vi "Force Channel Command.vi"(8 "error in":errorcluster, 10 "Channel Force Data":T1 {"Force Data" format="%x"}, 11 "CoreOOB_Rx in":refnum<class "CIFCoreOOB_Rx.lvclass">) -> (0 "error out":errorcluster, 3 "CoreOOB_Rx out":refnum<class "CIFCoreOOB_Rx.lvclass">)   [LabVIEW 2021, in "CIFCoreOOB_Rx.lvclass"]
uses:
  CIFCoreOOB_Rx.lvclass
  D:/dev/CIF-LVCore/src/CIFUtilities/CIFOutOfBand/CIFOutOfBand.lvclass
  Typedef/Channel Fault Data.ctl
  CIFUtilities/CIFOutOfBand/CIFOutOfBand.lvclass/CIFOutOfBand.ctl
  Typedef/OOB Core Commands.ctl
  Typedef/Template Payload.ctl
  Typedef/Channel Connection Data.ctl
  CIFCoreOOB_Rx.lvclass/CIFCoreOOB_Rx.ctl
  CIFUtilities/CIFOutOfBand/CIFOutOfBand.lvclass
  <vilib>/CIF Foundation/CIF Utilities/Time/Typedef/Timestamp Pair.ctl
  <vilib>/CIF Foundation/CIF Utilities/Time/Time_CIF_U.lvlib
  <vilib>/CIF Foundation/CIF Utilities/Time/Typedef/Clock Conversion Map.ctl
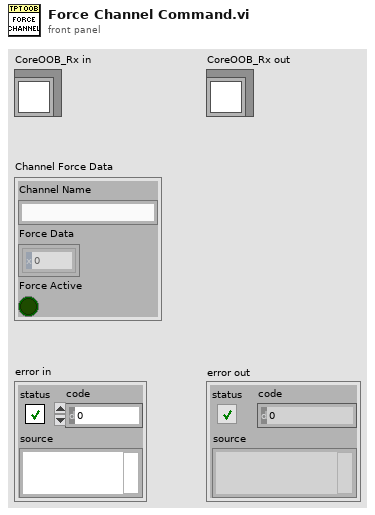
[diagram p1: front panel]
types:
  T1 = typedef "CIFCoreOOB_Rx.lvclass/Channel Fault Data.ctl" = cluster{"Channel Name":string, "Force Data":u8[], "Force Active":bool}
  T2 = typedef "CIFCoreOOB_Rx.lvclass/OOB Core Commands.ctl" = enum8{"Start", "Pause", "Stop", "RefreshStats", "UpdateConfig", "Connect Channel", "Force Channel", "Update Clock Map"}
  T3 = typedef "CIFCoreOOB_Rx.lvclass/Template Payload.ctl" = cluster{"Config Data":variant, "Connections":T4[], "Forces":T1[], "Clock Conversion":T5}
  T4 = typedef "CIFCoreOOB_Rx.lvclass/Channel Connection Data.ctl" = cluster{"Publisher Name":string, "Subscriber Name":string, "Connection Data":u8[]}
  T5 = typedef "Time_CIF_U.lvlib/Clock Conversion Map.ctl" = map{u8, cluster{"Last Reset":i64, "Offset Pair":T6, "Slope":dbl, "1/Slope":dbl}}
  T6 = typedef "Time_CIF_U.lvlib/Timestamp Pair.ctl" = cluster{"System Time":i64, "External Time":i64}
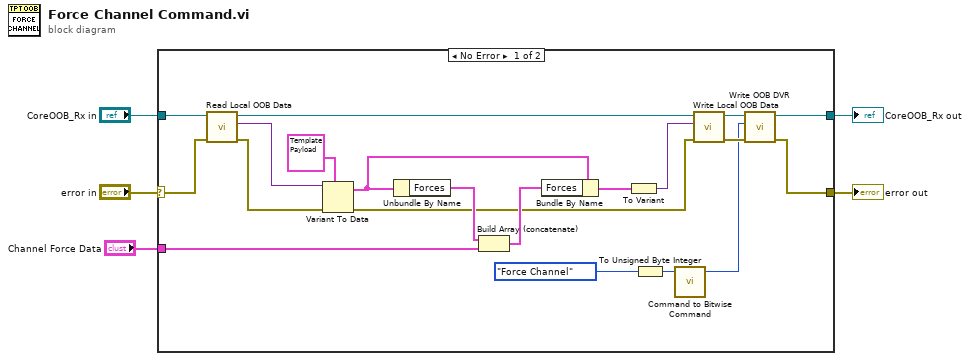
[diagram p0: block diagram]
diagram:
  n1 = case shown="No Error" "error in" {
    selector: "error in" -> [w21 w27]
    tunnel: [w24 w27] -> w4
    tunnel: "CoreOOB_Rx in" -> [w23 w26]
    tunnel: [w25 w26] -> w2
    tunnel: "Channel Force Data" -> [w8 _]
    frame No Error {
      n2 = call "Read Local OOB Data.vi"("error in"=w21, "OOB in"=w23) -> ("error out"=w17:errorcluster, "Local OOB Data"=w20:variant, "OOB out"=w22:refnum<class "CIFCoreOOB_Rx.lvclass">)  [unwired: 7 in]
      n3 = Variant To Data(error in=w17, type=T3 {"Config Data"=variant, "Connections"=[], "Forces"=[], "Clock Conversion"={}} ("Template Payload"), Variant=w20) -> (data=w18:T3, error out=w6:errorcluster)
      n4 = Unbundle By Name(w18) -> ("Forces"=w9:T1[])
      n5 = Build Array (concatenate)(w9, w8) -> (w7:T1[])
      n6 = Bundle By Name(cluster=w18, "Forces"=w7) -> (w12:T3)
      n7 = To Variant(anything=w12) -> (Variant=w11:variant)
      n8 = To Unsigned Byte Integer(number=OOB_Core_Commands."Force Channel" ("OOB Main Commands")) -> (unsigned 8bit integer=w14:u8)
      n9 = call "Command to Bitwise Command.vi"("OOB Command"=w14) -> ("bit command"=w10:u64)  [unwired: 3 in]
      n10 = call "Write Local OOB Data.vi"("error in"=w6, "Local OOB Data"=w11, "OOB in"=w22) -> ("error out"=w16:errorcluster, "OOB out"=w15:refnum<class "CIFCoreOOB_Rx.lvclass">)  [unwired: 7 in]
      n11 = call "Write OOB DVR.vi"("error in"=w16, "Commands (bitwise)"=w10, "OOB in"=w15) -> ("error out"=w24:errorcluster, "OOB out"=w25:refnum<class "CIFCoreOOB_Rx.lvclass">)  [unwired: 7 in]
    }
    frame Error {
    }
  }
  "error out" <- w4
  "CoreOOB_Rx out" <- w2
